vi "ClearInvader.vi"(8 "InvaderPosition":T1, 11 "IntensityArray_IN":u8[][](array[numeric])) -> (3 "IntensityArray_OUT":u8[][](array[numeric]))   [LabVIEW 2022 SP3]
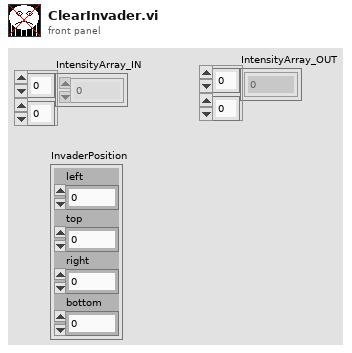
[diagram p1: front panel]
types:
  T1 = cluster{"left":i16, "top":i16, "right":i16, "bottom":i16}
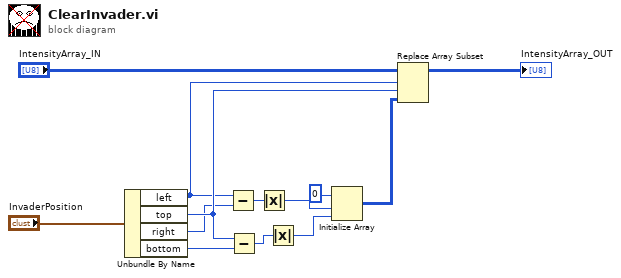
[diagram p0: block diagram]
diagram:
  n1 = Unbundle By Name("InvaderPosition") -> ("left"=w9:i16, "top"=w11:i16, "right"=w8:i16, "bottom"=w10:i16)
  n2 = Subtract(x=w9, y=w8) -> (x-y=w7:i16)
  n3 = Subtract(x=w11, y=w10) -> (x-y=w6:i16)
  n4 = Absolute Value(x=w7) -> (abs(x)=w4:i16)
  n5 = Absolute Value(x=w6) -> (abs(x)=w3:i16)
  n6 = Initialize Array(u8 0 ("element"), w4, w3) -> (w2:u8[][])
  n7 = Replace Array Subset(array="IntensityArray_IN", new element=w2, index (row)=w9, index (col)=w11) -> (→"IntensityArray_OUT":u8[][])
